vi "parse_start_points.vi"(4 "error in":errorcluster, 7 "Response":string) -> (0 "error out":errorcluster, 3 "Start locations":T1)   [LabVIEW 2019, in "Lib_Simx.lvlib"]
doc: "Parse the starting point information and generate a cluster with the coordinates of each point and the type. If a point is PIE type, it will be move to the top of the list. The PIE point is the camera position."
uses:
  Lib_Simx.lvlib
  controls/start_points.ctl
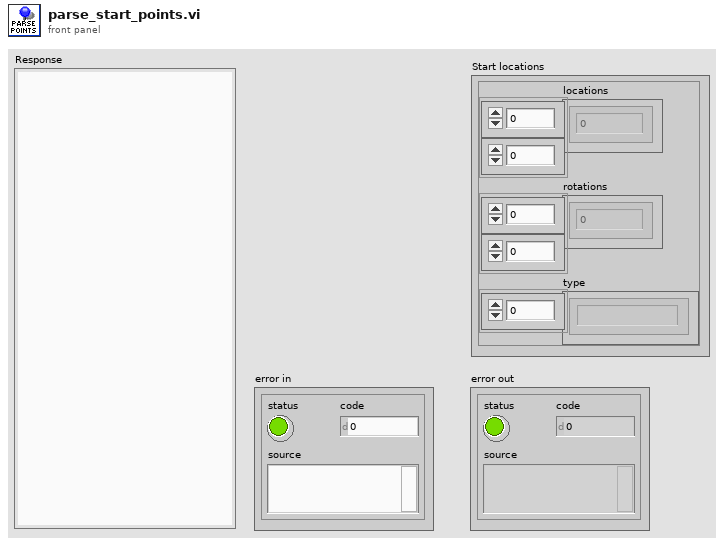
[diagram p1: front panel]
types:
  T1 = cluster{"locations":dbl[][], "rotations":dbl[][], "type":string[]}
  T2 = typedef "Lib_Simx.lvlib/start_points.ctl" = cluster{"locations":dbl[][], "rotations":dbl[][], "type":string[]}
  T3 = cluster{"reference":dbl, "success":bool, "type":string, "message":string}
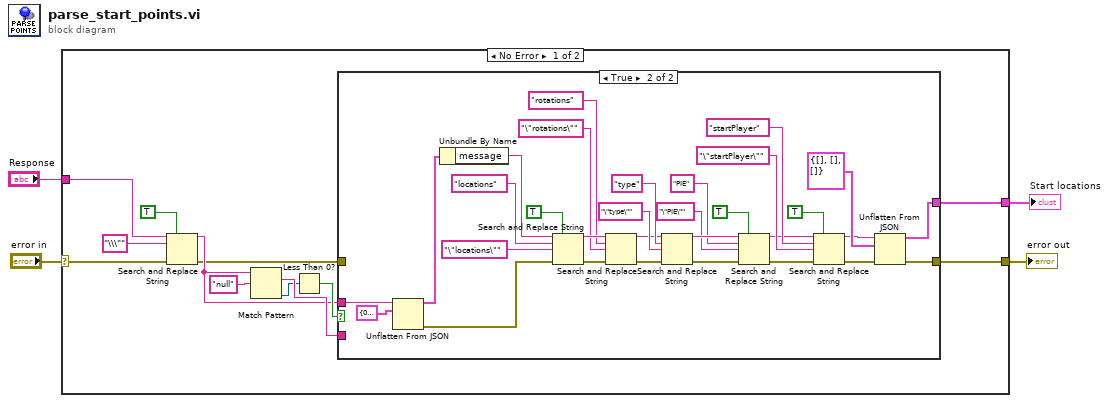
[diagram p0: block diagram]
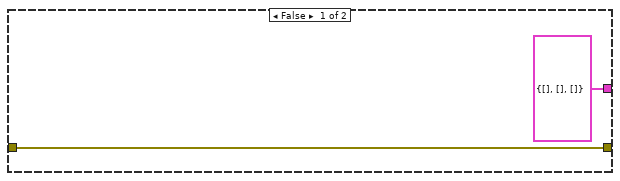
[diagram p2: hidden frame]
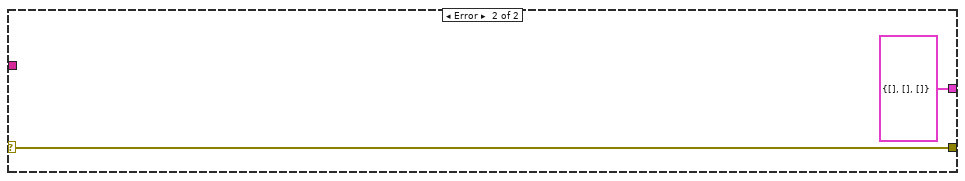
[diagram p3: hidden frame]
diagram:
  n1 = case shown="No Error" "error in" {
    selector: "error in" -> [w14 w51]
    tunnel: [w13 w51] -> w3
    tunnel: [w6 T1 {"locations"=[], "rotations"=[], "type"=[]} ("message")] -> w2
    tunnel: "Response" -> [w5 _]
    frame No Error {
      n2 = Search and Replace String(replace all?=TRUE ("replace all? (F)"), input string=w5, search string="\\\"", error in=w14) -> (result string=w8:string, error out=w7:errorcluster)  [unwired: 4 in, 2 out]
      n3 = Match Pattern(string=w8, regular expression="null") -> (match substring=w12:string, offset past match=w10:i32)  [unwired: 1 in, 2 out]
      n4 = Less Than 0?(x=w10) -> (x < 0?=w9:bool)
      n5 = case shown="True" w9 {
        tunnel: w8 -> [_ w49]
        tunnel: w12 -> [_ _]
        tunnel: [w18 w39] -> w13
        tunnel: w7 -> [w18 _]
        tunnel: [T1 {"locations"=[], "rotations"=[], "type"=[]} ("message") w33] -> w6
        frame False {
        }
        frame True {
          n6 = Unflatten From JSON(JSON string=w49, type and defaults=T3 {"reference"=0.0, "success"=TRUE, "type"="", "message"=""}) -> (value=w47:T3, error out=w38:errorcluster)  [unwired: 5 in]
          n7 = Unbundle By Name(w47) -> ("message"=w46:string)
          n8 = Search and Replace String(replace all?=TRUE ("replace all? (F)"), input string=w46, search string="locations" ("replace string (\"\")"), replace string="\"locations\"" ("replace string (\"\")"), error in=w38) -> (result string=w42:string, error out=w37:errorcluster)  [unwired: 3 in, 2 out]
          n9 = Search and Replace String(input string=w42, search string="rotations" ("replace string (\"\")"), replace string="\"rotations\"" ("replace string (\"\")"), error in=w37) -> (result string=w31:string, error out=w32:errorcluster)  [unwired: 4 in, 2 out]
          n10 = Search and Replace String(input string=w31, search string="type" ("replace string (\"\")"), replace string="\"type\"" ("replace string (\"\")"), error in=w32) -> (result string=w29:string, error out=w30:errorcluster)  [unwired: 4 in, 2 out]
          n11 = Search and Replace String(replace all?=TRUE ("replace all? (F)"), input string=w29, search string="PIE", replace string="\"PIE\"" ("replace string (\"\")"), error in=w30) -> (result string=w22:string, error out=w26:errorcluster)  [unwired: 3 in, 2 out]
          n12 = Search and Replace String(replace all?=TRUE ("replace all? (F)"), input string=w22, search string="startPlayer" ("input string"), replace string="\"startPlayer\"" ("search string"), error in=w26) -> (result string=w21:string, error out=w25:errorcluster)  [unwired: 3 in, 2 out]
          n13 = Unflatten From JSON(JSON string=w21, type and defaults=T2 {"locations"=[], "rotations"=[], "type"=[]} ("message"), error in (no error)=w25) -> (value=w33:T2, error out=w39:errorcluster)  [unwired: 4 in]
        }
      }
    }
    frame Error {
    }
  }
  "error out" <- w3
  "Start locations" <- w2
